vi "_TBD Timestamp to Datetime String.vi"(1 "Timestamp":timestamp) -> (0 "Date-Time String":string)   [LabVIEW 2023, in "Error Manager.lvlib" / "Error Log.lvclass"]
uses:
  Error Log.lvclass
  Error Log.lvclass/Error Log.ctl
panel:
  # "Input\nInputs to the VI"
  # "Development\nControls or indicators that are useful for development or testing, but which are not outputs of the VI."
  # "Output\nOutputs of the VI"
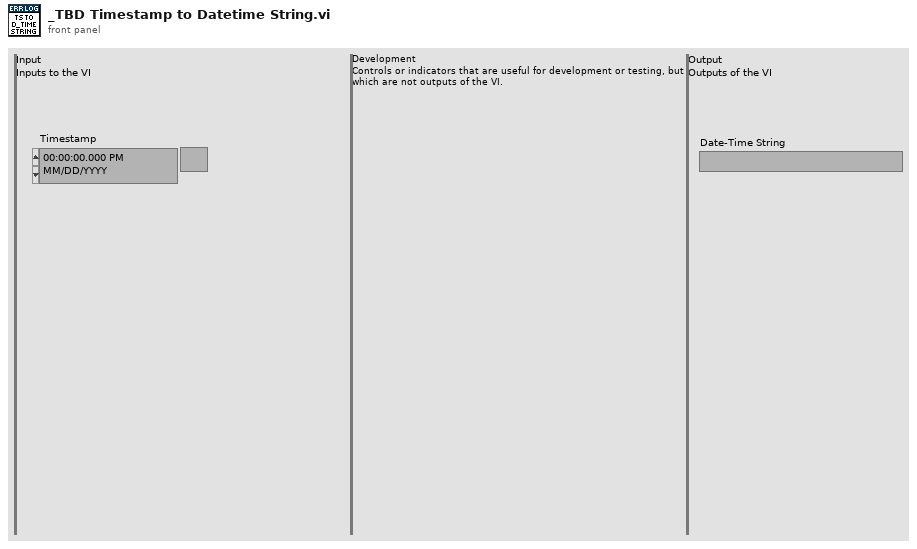
[diagram p1: front panel]
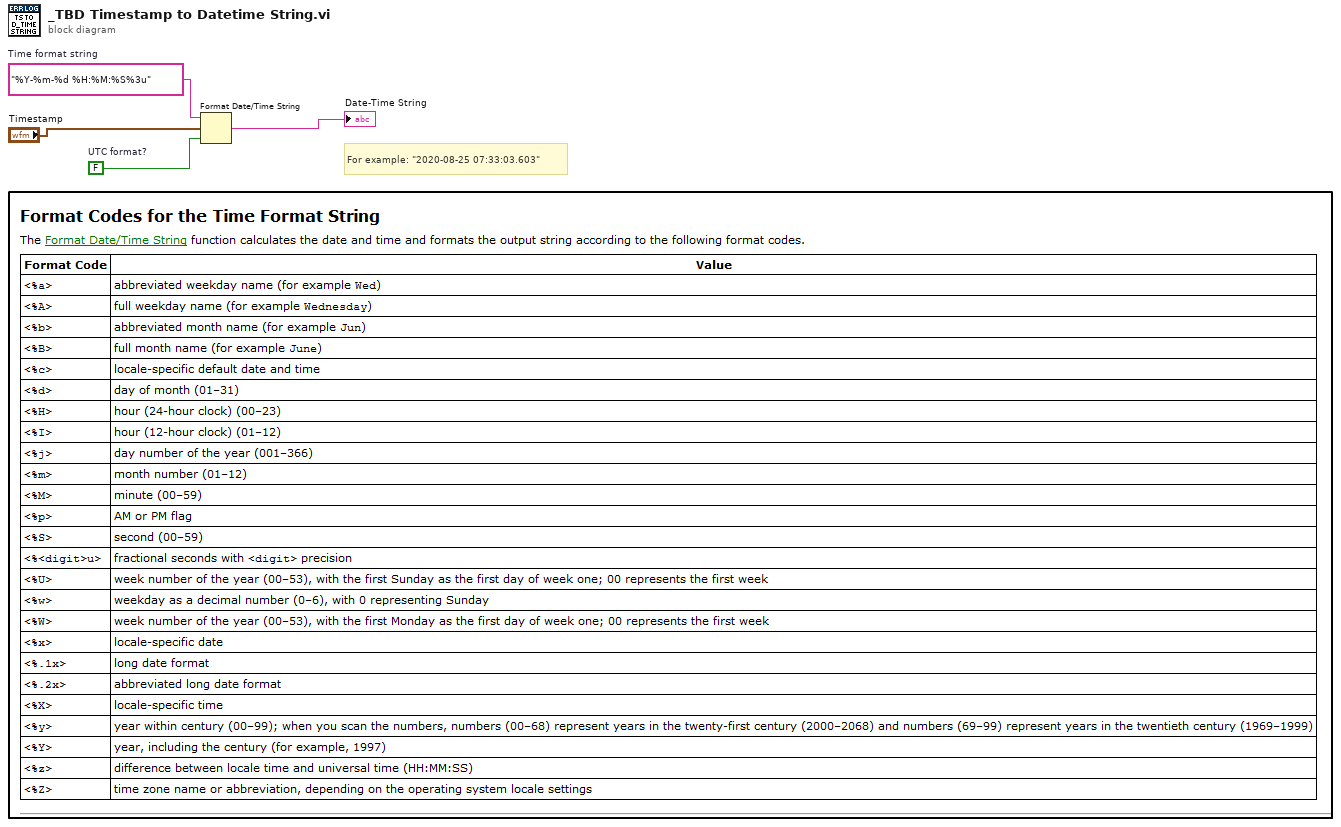
[diagram p0: block diagram]
diagram:
  w1 = FALSE  # UTC format?
  w4 = "%Y-%m-%d %H:%M:%S%3u"  # Time format string
  # "For example: \"2020-08-25 07:33:03.603\""
  n1 = Format Date/Time String(time format string (%c)=w4, seconds (now)="Timestamp", UTC format=w1) -> (date/time string=→"Date-Time String":string)
